vi "SetupSweepAndGetPeak.vi"(6 "Route Names":string[](array[string]), 7 "Cal?":bool, 8 "error in (no error)":errorcluster, 9 "Span(Hz)":dbl=26500000000.0, 10 "Center Frequency(Hz)":dbl=13250000000.0, 11 "SpecA_MXA in":refnum<class "SpecA_MXA.lvclass">) -> (0 "error out":errorcluster, 1 "FDelta(hz)":dbl, 2 "RSL (dBm)":dbl, 3 "SpecA_MXA out":refnum<class "SpecA_MXA.lvclass">)   [LabVIEW 2014, in "SpecA_MXA.lvclass"]
uses:
  SpecA_MXA.lvclass
  SpecA_MXA.lvclass/SpecA_MXA.ctl
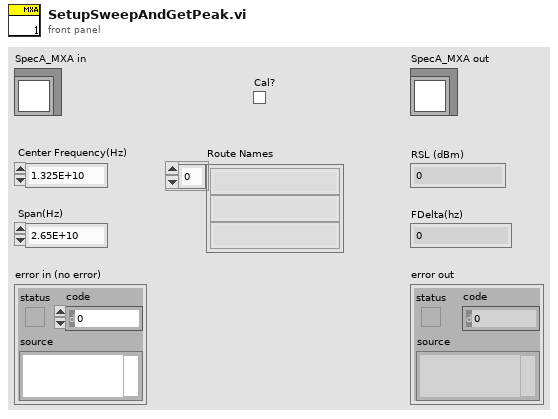
[diagram p1: front panel]
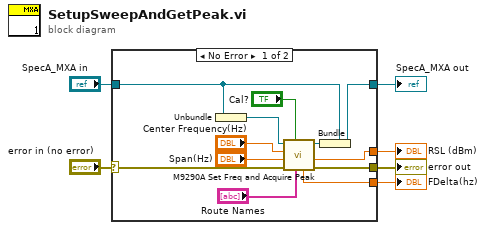
[diagram p0: block diagram]
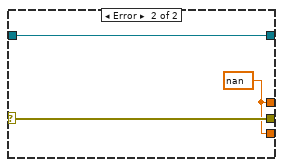
[diagram p2: hidden frame]
diagram:
  n1 = case shown="No Error" "error in (no error)" {
    selector: "error in (no error)" -> [w10 w20]
    tunnel: "SpecA_MXA in" -> [w13 w21]
    tunnel: [w14 w21] -> w4
    tunnel: [w12 w19] -> w3
    tunnel: [w11 w19] -> w2
    tunnel: [w9 w20] -> w1
    frame No Error {
      n2 = Unbundle(w13) -> (w16:refnum<visa-resource-name>)
      n3 = call "M9290A Set Freq and Acquire Peak.vi"("Route Names"="Route Names", "Cal?"="Cal?", "error in (no error)"=w10, "Span(Hz)"="Span(Hz)", "Center Frequency(Hz)"="Center Frequency(Hz)", "VISA resource name"=w16) -> ("error out"=w9:errorcluster, "Amplitude (Cal)"=w12:dbl, "VISA out"=w15:refnum<visa-resource-name>, "FDelta"=w11:dbl)  [unwired: 1 in, 1 out]
      n4 = Bundle(cluster=w13, w15) -> (w14:refnum<class "SpecA_MXA.lvclass">)
    }
    frame Error {
      w19 = nan ("Amplitude (Cal)")
    }
  }
  "error out" <- w1
  "SpecA_MXA out" <- w4
  "FDelta(hz)" <- w2
  "RSL (dBm)" <- w3
